vi "Reset.vi"(8 "error in (no error)":errorcluster, 11 "RMX4120 in":refnum<class "RMX4120.lvclass">) -> (0 "error out":errorcluster, 3 "RMX4120 out":refnum<class "RMX4120.lvclass">)   [LabVIEW 2023, in "RMX4120.lvclass"]
uses:
  RMX4120.lvclass
  RMXPowerSupply.lvclass
  RMX4120.lvclass/RMX4120.ctl
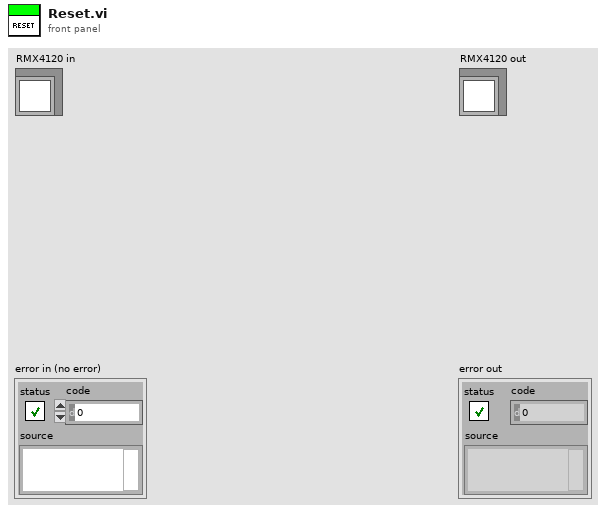
[diagram p1: front panel]
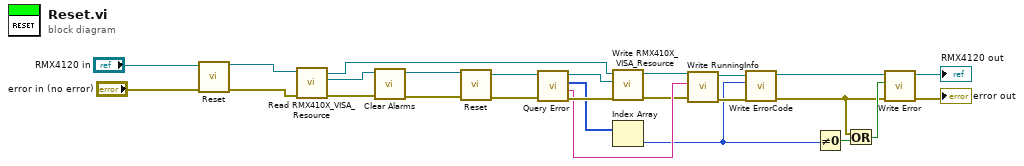
[diagram p0: block diagram]
diagram:
  n1 = call-parent "Reset.vi"("error in (no error)"="error in (no error)", "RMXPowerSupply in"="RMX4120 in") -> ("error out"=w21:errorcluster, "RMXPowerSupply out"=w19:refnum<class "RMX4120.lvclass">)  [unwired: 8 in]
  n2 = call-dynamic "Read RMX410X_VISA_Resource.vi"("error in (no error)"=w21, "RMXPowerSupply in"=w19) -> ("error out"=w20:errorcluster, "RMX410X_VISA_Resource"=w18:refnum<visa-resource-name>, "RMXPowerSupply out"=w14:refnum<class "RMX4120.lvclass">)  [unwired: 7 in]
  n3 = call "Clear Alarms.vi"("error in (no error)"=w20, "VISA resource name"=w18) -> ("error out"=w24:errorcluster, "VISA resource name out"=w17:refnum<visa-resource-name>)  [unwired: 8 in]
  n4 = call "Reset.vi"("error in (no error)"=w24, "VISA resource name"=w17) -> ("error out"=w23:errorcluster, "VISA resource name out"=w16:refnum<visa-resource-name>)  [unwired: 8 in]
  n5 = call "Query Error.vi"("error in (no error)"=w23, "VISA resource name"=w16) -> ("error out"=w22:errorcluster, "Error Message"=w13:string, "Error Code"=w12:i32[], "VISA resource name out"=w15:refnum<visa-resource-name>)  [unwired: 6 in]
  n6 = call-dynamic "Write RMX410X_VISA_Resource.vi"("error in (no error)"=w22, "RMX410X_VISA_Resource"=w15, "RMXPowerSupply in"=w14) -> ("error out"=w11:errorcluster, "RMXPowerSupply out"=w9:refnum<class "RMX4120.lvclass">)  [unwired: 7 in]
  n7 = Index Array(array=w12) -> (element=w7:i32)  [unwired: 1 in]
  n8 = call-dynamic "Write RunningInfo.vi"("error in (no error)"=w11, "RunningInfo"=w13, "RMXPowerSupply in"=w9) -> ("error out"=w10:errorcluster, "RMXPowerSupply out"=w8:refnum<class "RMX4120.lvclass">)  [unwired: 7 in]
  n9 = call-dynamic "Write ErrorCode.vi"("error in (no error)"=w10, "ErrorCode"=w7, "RMXPowerSupply in"=w8) -> ("error out"=w3:errorcluster, "RMXPowerSupply out"=w2:refnum<class "RMX4120.lvclass">)  [unwired: 7 in]
  n10 = Not Equal To 0?(x=w7) -> (x != 0?=w6:bool)
  n11 = Or(x=w3, y=w6) -> (x .or. y?=w5:bool)
  n12 = call-dynamic "Write Error.vi"("error in (no error)"=w3, "Error"=w5, "RMXPowerSupply in"=w2) -> ("error out"=→"error out":errorcluster, "RMXPowerSupply out"=→"RMX4120 out":refnum<class "RMX4120.lvclass">)  [unwired: 7 in]
